vi "Swerve Drive.vi"(0 "X":dbl, 1 "Rot. Point X":dbl, 3 "Rot. Point Y":dbl, 5 "Y":dbl, 7 "Z":dbl, 11 "Error In":errorcluster, 12 "Robot Centric?":bool=TRUE, 13 "Autonomous?":bool, 14 "Yaw":dbl) -> (4 "Front Left Output":dbl, 6 "Front Right Output":dbl, 8 "Back Left Output":dbl, 10 "Back Right Output":dbl, 15 "Error Out":errorcluster)   [LabVIEW 2017]
uses:
  Public/Documents/Cross The Road Electronics/Phoenix-LabVIEW/Motor Controller/Controls/CTRE_Phoenix_MotorControl_ControlMode.ctl
  <vilib>/Rock Robotics/Network Tables/NT Read Number.vi
  <vilib>/Rock Robotics/Network Tables/NT Write Numeric Array.vi
panel:
  in  "Robot Length":dbl=33.5
  in  "Robot Width":dbl=28.5
  # "Swerve Drive Teleoperated Control\nFRC Team 34"
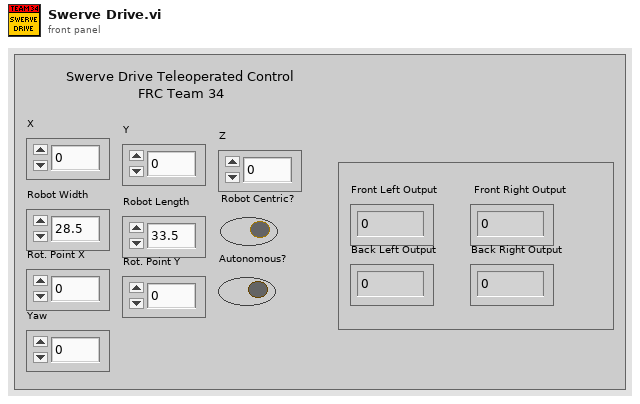
[diagram p1: front panel]
types:
  T1 = typedef "CTRE_Phoenix_MotorControl_ControlMode.ctl" = u16
  T2 = enum16{"Front Left", "Front Right", "Back Left", "Back Right"}
  T3 = typedef "WPI_MotorControlDeviceRef.ctl" = cluster{"DeviceStatus":errorcluster, "Type":T4, "PWM":cluster{"PWM Channel":T5, "DeadBand":T6}, "CAN":cluster{"Device Number":u8, "SetOutput VI Ref":variant, "GetOutput VI Ref":variant, "Enable VI Ref":variant, "Disable VI Ref":variant, "Data":variant}, "Invert":bool, "DIO PWM":cluster{"PWM \"Enable\" Channel":T5, "DIOChannel":T7, "PWM Rate":dbl}}
  T4 = typedef "WPI_MotorControlType.ctl" = enum16{"PWM", "CAN", "DIO PWM"}
  T5 = typedef "FPGA_DIOPWMChannel.ctl" = enum8{"PWM 0", "PWM 1", "PWM 2", "PWM 3", "PWM 4", "PWM 5", "PWM 6", "PWM 7", "PWM 8", "PWM 9", "PWM MXP 0", "PWM MXP 1", "PWM MXP 2", "PWM MXP 3", "PWM MXP 4", "PWM MXP 5", "PWM MXP 6", "PWM MXP 7", "PWM MXP 8", "PWM MXP 9", "Invalid"}
  T6 = typedef "WPI_PWMDeadband.ctl" = cluster{"Name":string, "maxPositivePwm":i32, "minPositivePwm":i32, "centerPwm":i32, "maxNegativePwm":i32, "minNegativePwm":i32, "angularRange":u16}
  T7 = typedef "FPGA_DIOChannel.ctl" = enum8{"DIO 0", "DIO 1", "DIO 2", "DIO 3", "DIO 4", "DIO 5", "DIO 6", "DIO 7", "DIO 8", "DIO 9", "DIO MXP 0", "DIO MXP 1", "DIO MXP 2", "DIO MXP 3", "DIO MXP 4", "DIO MXP 5", "DIO MXP 6", "DIO MXP 7", "DIO MXP 8", "DIO MXP 9", "DIO MXP 10", "DIO MXP 11", "DIO MXP 12", "DIO MXP 13", "DIO MXP 14", "DIO MXP 15", "SPI Port CS1", "SPI Port CS2", "SPI Port CS3", "SPI Port MISO", "SPI Port MOSI", "Invalid"}
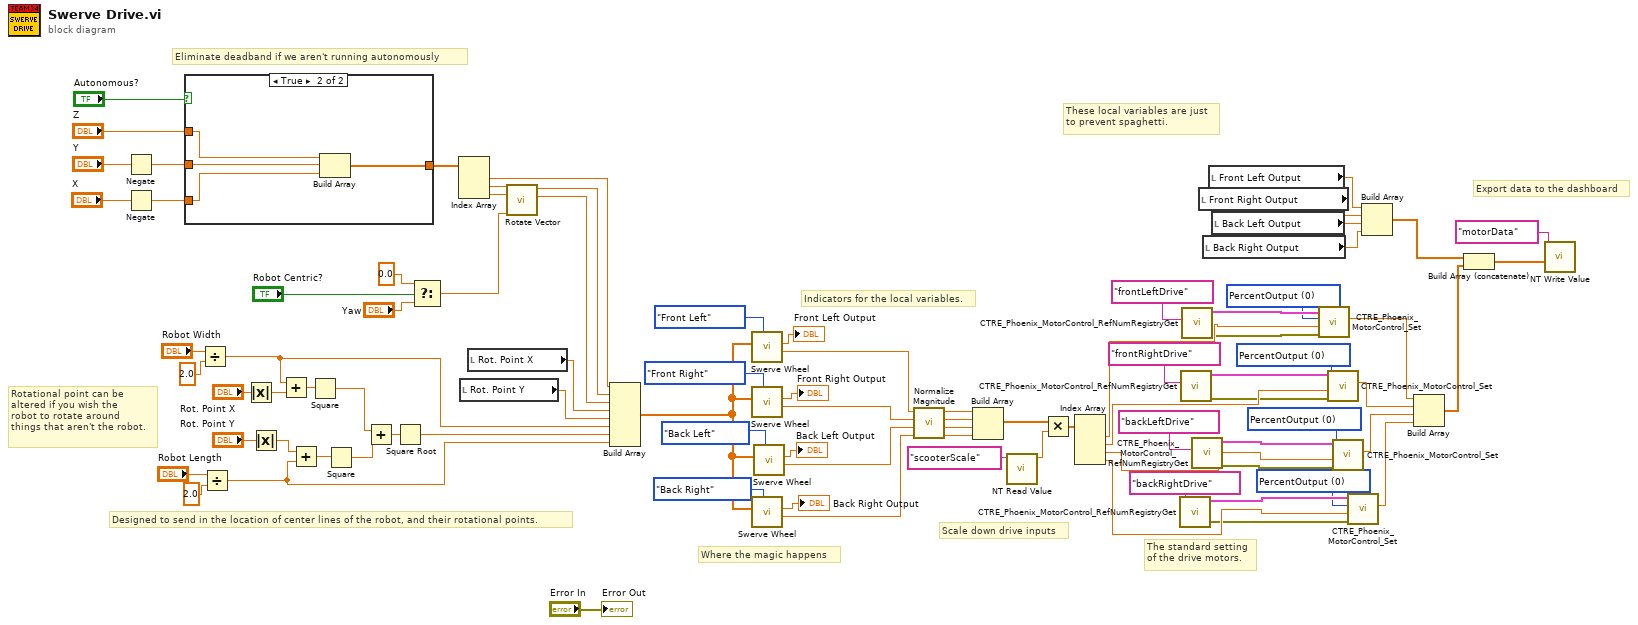
[diagram p0: block diagram]
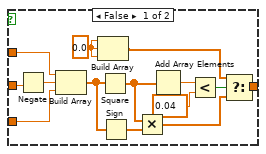
[diagram p2: hidden frame]
diagram:
  w13 = T1 0 items=["PercentOutput"=0, "Position"=1, "Velocity"=2, "Current"=3, "Follower"=5, "MotionProfile"=6, "MotionMagic"=7, "MotionMagicArc"=8, "MotionProfileArc"=10, "Disabled"=15] ("Control Mode")
  w14 = T1 0 items=["PercentOutput"=0, "Position"=1, "Velocity"=2, "Current"=3, "Follower"=5, "MotionProfile"=6, "MotionMagic"=7, "MotionMagicArc"=8, "MotionProfileArc"=10, "Disabled"=15] ("Control Mode")
  w15 = T1 0 items=["PercentOutput"=0, "Position"=1, "Velocity"=2, "Current"=3, "Follower"=5, "MotionProfile"=6, "MotionMagic"=7, "MotionMagicArc"=8, "MotionProfileArc"=10, "Disabled"=15] ("Control Mode")
  w16 = T1 0 items=["PercentOutput"=0, "Position"=1, "Velocity"=2, "Current"=3, "Follower"=5, "MotionProfile"=6, "MotionMagic"=7, "MotionMagicArc"=8, "MotionProfileArc"=10, "Disabled"=15] ("Control Mode")
  # "Export data to the dashboard"
  # "Indicators for the local variables."
  # "Rotational point can be \naltered if you wish the \nrobot to rotate around \nthings that aren't the robot."
  # "Scale down drive inputs"
  # "Eliminate deadband if we aren't running autonomously"
  # "These local variables are just \nto prevent spaghetti."
  # "Where the magic happens"
  # "The standard setting\nof the drive motors."
  # "Designed to send in the location of center lines of the robot, and their rotational points."
  n1 = Negate(x="Y") -> (-x=w34:dbl)
  n2 = Negate(x="X") -> (-x=w33:dbl)
  n3 = case shown="True" "Autonomous?" {
    tunnel: w34 -> [w92 w105]
    tunnel: [w91 w103] -> w87
    tunnel: "Z" -> [w90 w106]
    tunnel: w33 -> [w89 w104]
    frame False {
      w98 = 0.0 ("element")
      n4 = Negate(x=w92) -> (-x=w94:dbl)
      n5 = Build Array(w90, w94, w89) -> (w97:dbl[])
      n6 = Build Array(w98, w98, w98) -> (w99:dbl[])
      n7 = Square(x=w97) -> (x^2=w95:dbl[])
      n8 = Sign(1:w97) -> (0:w96:dbl[])
      n9 = Multiply(x=w95, y=w96) -> (x*y=w93:dbl[])
      n10 = Add Array Elements(numeric array=w95) -> (sum=w102:dbl)
      n11 = Less?(x=w102, y=0.04 ("x")) -> (x < y?=w100:bool)
      n12 = Select(t=w99, s=w100, f=w93) -> (s? t:f=w91:dbl[])
    }
    frame True {
      n13 = Build Array(w106, w105, w104) -> (w103:dbl[])
    }
  }
  n14 = Divide(x="Robot Width", y=2.0) -> (x/y=w61:dbl)
  n15 = Divide(x="Robot Length", y=2.0) -> (x/y=w59:dbl)
  n16 = Absolute Value(x="Rot. Point X") -> (abs(x)=w73:dbl)
  n17 = Absolute Value(x="Rot. Point Y") -> (abs(x)=w70:dbl)
  n18 = Add(x=w61, y=w73) -> (x+y=w72:dbl)
  n19 = Add(x=w70, y=w59) -> (x+y=w71:dbl)
  n20 = Square(x=w72) -> (x^2=w68:dbl)
  n21 = Square(x=w71) -> (x^2=w69:dbl)
  n22 = Add(x=w68, y=w69) -> (x+y=w67:dbl)
  n23 = Square Root(x=w67) -> (sqrt(x)=w60:dbl)
  n24 = Select(t=0.0, s="Robot Centric?", f="Yaw") -> (s? t:f=w80:dbl)
  n25 = Index Array(array=w87) -> (element #1=w66:dbl, element #2=w82:dbl, element #3=w81:dbl)  [unwired: 3 in]
  n26 = local read "Rot. Point Y"() -> (w62:dbl)
  n27 = local read "Rot. Point X"() -> (w63:dbl)
  n28 = call "Rotate Vector.vi"("Angle"=w80, "X"=w81, "Y"=w82) -> ("X'"=w64:dbl, "Y'"=w65:dbl)  [unwired: 7 in]
  n29 = Build Array(w66, w65, w64, w63, w62, w61, w60, w59) -> (w58:dbl[])
  n30 = call "Swerve Wheel.vi"("Wheel"=T2."Front Left", "Inputs"=w58) -> ("Speed"=w53:dbl, "Motor Output"=→"Front Left Output":dbl)  [unwired: 8 in]
  n31 = call "Swerve Wheel.vi"("Wheel"=T2."Front Right", "Inputs"=w58) -> ("Speed"=w52:dbl, "Motor Output"=→"Front Right Output":dbl)  [unwired: 8 in]
  n32 = call "Swerve Wheel.vi"("Wheel"=T2."Back Right", "Inputs"=w58) -> ("Speed"=w50:dbl, "Motor Output"=→"Back Right Output":dbl)  [unwired: 8 in]
  n33 = call "Swerve Wheel.vi"("Wheel"=T2."Back Left", "Inputs"=w58) -> ("Speed"=w51:dbl, "Motor Output"=→"Back Left Output":dbl)  [unwired: 8 in]
  n34 = call "Normalize Magnitude.vi"("D"=w50, "C"=w51, "B"=w52, "A"=w53) -> ("D'"=w46:dbl, "C'"=w47:dbl, "B'"=w48:dbl, "A'"=w49:dbl)  [unwired: 4 in]
  n35 = Build Array(w49, w48, w47, w46) -> (w45:dbl[])
  n36 = call-poly <vilib>:"NT Read Value.vi"("Name"="scooterScale") -> ("Numeric"=w43:dbl)  [unwired: 9 in, 1 out]
  n37 = Multiply(x=w45, y=w43) -> (x*y=w42:dbl[])
  n38 = Index Array(array=w42) -> (element #1=w27:dbl, element #2=w21:dbl, element #3=w18:dbl, element #4=w24:dbl)  [unwired: 4 in]
  n39 = call "CTRE_Phoenix_MotorControl_RefNumRegistryGet.vi"("refnum name"="backRightDrive") -> ("error out"=w23:errorcluster, "PhoenixMotorControlDevRef"=w25:T3)  [unwired: 9 in]
  n40 = call "CTRE_Phoenix_MotorControl_RefNumRegistryGet.vi"("refnum name"="frontRightDrive") -> ("error out"=w20:errorcluster, "PhoenixMotorControlDevRef"=w22:T3)  [unwired: 9 in]
  n41 = call "CTRE_Phoenix_MotorControl_RefNumRegistryGet.vi"("refnum name"="frontLeftDrive") -> ("error out"=w26:errorcluster, "PhoenixMotorControlDevRef"=w28:T3)  [unwired: 9 in]
  n42 = call "CTRE_Phoenix_MotorControl_RefNumRegistryGet.vi"("refnum name"="backLeftDrive") -> ("error out"=w17:errorcluster, "PhoenixMotorControlDevRef"=w19:T3)  [unwired: 9 in]
  n43 = local read "Front Right Output"() -> (w8:dbl)
  n44 = local read "Back Right Output"() -> (w6:dbl)
  n45 = local read "Front Left Output"() -> (w9:dbl)
  n46 = local read "Back Left Output"() -> (w7:dbl)
  n47 = call "CTRE_Phoenix_MotorControl_Set.vi"("error in (no error)"=w26, "Output"=w27, "Control Mode"=w16, "PhoenixMotorControlDevRef"=w28) -> ("Motor Output"=w5:dbl)  [unwired: 5 in, 2 out]
  n48 = call "CTRE_Phoenix_MotorControl_Set.vi"("error in (no error)"=w20, "Output"=w21, "Control Mode"=w15, "PhoenixMotorControlDevRef"=w22) -> ("Motor Output"=w4:dbl)  [unwired: 5 in, 2 out]
  n49 = call "CTRE_Phoenix_MotorControl_Set.vi"("error in (no error)"=w17, "Output"=w18, "Control Mode"=w14, "PhoenixMotorControlDevRef"=w19) -> ("Motor Output"=w3:dbl)  [unwired: 5 in, 2 out]
  n50 = call "CTRE_Phoenix_MotorControl_Set.vi"("error in (no error)"=w23, "Output"=w24, "Control Mode"=w13, "PhoenixMotorControlDevRef"=w25) -> ("Motor Output"=w2:dbl)  [unwired: 5 in, 2 out]
  n51 = Build Array(w9, w8, w7, w6) -> (w12:dbl[])
  n52 = Build Array(w5, w4, w3, w2) -> (w1:dbl[])
  n53 = Build Array (concatenate)(w12, w1) -> (w11:dbl[])
  n54 = call-poly <vilib>:"NT Write Value.vi"("Numeric Array"=w11, "Name"="motorData") -> ()  [unwired: 9 in, 1 out]
  "Error Out" <- "Error In"
